vi "cw_5_2.vi"() -> ()   [LabVIEW 2022 SP3]
uses:
  <vilib>/numeric/Random Number (Range) DBL.vi
  <vilib>/Utility/file.llb/Write Delimited Spreadsheet (string).vi
panel:
  out "error out":errorcluster
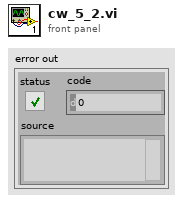
[diagram p1: front panel]
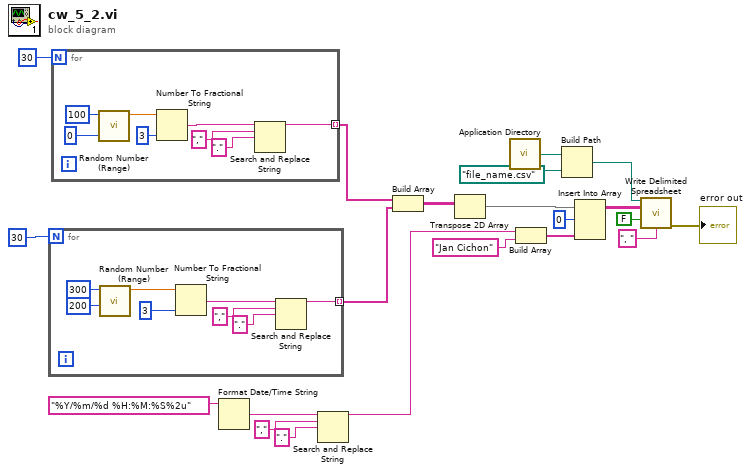
[diagram p0: block diagram]
diagram:
  n1 = for {
    N: 30 -> [_]
    tunnel: [w22] -> w17 mode=indexing
    n2 = call-poly <vilib>:"Random Number (Range).vi"("lower bound (0)"=u64 200, "upper bound (100)"=u64 300) -> ("number"=w26:dbl)  [unwired: 9 in]
    n3 = Number To Fractional String(number=w26, precision (6)=i16 3 ("width (-)")) -> (F-format string=w23:string)  [unwired: 2 in]
    n4 = Search and Replace String(input string=w23, search string=",", replace string="." ("replace string (\"\")")) -> (result string=w22:string)  [unwired: 5 in, 3 out]
  }
  n5 = for {
    N: 30 -> [_]
    tunnel: [w30] -> w18 mode=indexing
    n6 = call-poly <vilib>:"Random Number (Range).vi"("lower bound (0)"=u64 0, "upper bound (100)"=u64 100) -> ("number"=w35:dbl)  [unwired: 9 in]
    n7 = Number To Fractional String(number=w35, precision (6)=i16 3 ("width (-)")) -> (F-format string=w33:string)  [unwired: 2 in]
    n8 = Search and Replace String(input string=w33, search string=",", replace string="." ("replace string (\"\")")) -> (result string=w30:string)  [unwired: 5 in, 3 out]
  }
  n9 = Format Date/Time String(time format string (%c)="%Y/%m/%d %H:%M:%S%2u") -> (date/time string=w9:string)  [unwired: 2 in]
  n10 = Search and Replace String(input string=w9, search string=",", replace string="." ("replace string (\"\")")) -> (result string=w8:string)  [unwired: 5 in, 3 out]
  n11 = Build Array(w18, w17) -> (w19:string[][])
  n12 = Transpose 2D Array(2D array=w19) -> (transposed array=w15:string[][])
  n13 = call <vilib>:"Application Directory.vi"() -> ("Application Directory"=w6:path)
  n14 = Build Array(w8, "Jan Cichon") -> (w14:string[])
  n15 = Build Path(base path=w6, name or relative path=path "file_name.csv") -> (appended path=w4:path)
  n16 = Insert Into Array(array=w15, index (row)=0, new element=w14) -> (w7:string[][])  [unwired: 1 in]
  n17 = call-poly <vilib>:"Write Delimited Spreadsheet.vi"("file path (dialog if empty)"=w4, "2D data"=w7, "append to file? (new file:F)"=FALSE, "delimiter (\\t)"=", " ("delimiter (\\t)")) -> ("error out"=→"error out":errorcluster)  [unwired: 10 in, 1 out]
